vi "FPGA-Main.vi"() -> ()   [LabVIEW 2019]
uses:
  <vilib>/rvi/Emulation/niFpgaGetClockAttributes.vi
  <vilib>/rvi/Emulation/niFpgaSctlEmulationGetInTimedLoop.vi
  <vilib>/rvi/Emulation/niFpgaEmulationReportErrorSimple.vi
  <vilib>/rvi/eio/common/nirviEmuTemplateMethod_errors.vi
  <vilib>/rvi/Emulation/niFpgaEmulationIsFPGAContextNoSignature.vi
  <vilib>/rvi/errors/niFpgaSetErrorForExecOnDevCompSimple.vi
  <vilib>/rvi/eio/common/nirviEmuReportErrorAndStop.vi
  <vilib>/rvi/DataTransferAndStorage/Container/Common/niFpgaContainerGetUniqueNameForEmu.vi
  <vilib>/rvi/FIFO/Fifo_Resource/nirvififoEmulationSetSize.vi
  <vilib>/rvi/FIFO/Fifo_Resource/nirviFifoEmulationQueueMgr.vi
  <instcachedir>/0/nirviFifoEmulationQueueMgr_E5CAEC123FF24DC58D834DCA3CDAA9B5.lvgen/nirviFifoEmulationQueueMgr_E5CAEC123FF24DC58D834DCA3CDAA9B5_006.vi
  <vilib>/rvi/FIFO/Fifo_Resource/nirvififoEmulationDetermineInputValidOut.vi
  <vilib>/rvi/FIFO/Fifo_Resource/nirvififoEmulationCreateLock.vi
  <vilib>/rvi/Emulation/niFpgaProcessEmulError.vi
  <vilib>/rvi/FIFO/Fifo_Resource/nirvififoEmulationObtainLock.vi
  <vilib>/rvi/FIFO/Fifo_Resource/nirvififoEmulationReleaseLock.vi
  <vilib>/rvi/occurrence/nirviWaitOnOccurrenceBase.vi
  <vilib>/rvi/errors/nirviReportUnexpectedCaseInternalError.vi
  <vilib>/rvi/errors/nirviReportUnexpectedCaseInternalError (U32).vi
  <vilib>/rvi/Emulation/niFpgaCriticalErrorInLSC.vi
  <vilib>/Utility/error.llb/Clear Errors.vi
  <vilib>/rvi/interface/RandomDataEmulation/niFpgaRandomDataHandleErrors.vi
  <vilib>/rvi/interface/RandomDataEmulation/nirviRandomDataMultiElementFPGAFIFO.vi
  <instcachedir>/0/nirviRandomDataMultiElementFPGAFIFO_1ED88BA00AC641F388A9B1FAA20E354D.lvgen/nirviRandomDataMultiElementFPGAFIFO_1ED88BA00AC641F388A9B1FAA20E354D_004.vi
  <vilib>/eio/EIONode/EIONode.xnode
  <vilib>/rvi/DataTransferAndStorage/Container/XNode/niFpgaContainer.xnode
  <vilib>/rvi/FIFO/Fifo_Resource/nirvififoEmulationWrite.vi
  <vilib>/rvi/FIFO/Fifo_Resource/nirvififoEmulationRead.vi
  <vilib>/rvi/interface/RandomDataEmulation/nirviRandomDataFpgaReadWriteTemplate.vi
  <vilib>/rvi/Analysis/measure/butterworth/XNode/niFpgaButterworthFilter.xnode
  <vilib>/rvi/interface/RandomDataEmulation/nirviRandomDataFpgaMultiElementTemplate.vi
panel:
  out "超时？ 2":bool
  out "超时？":bool
  in  "Count(uSec)":u32=10 caption="计数器(uSec)"
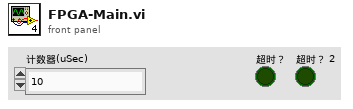
[diagram p1: front panel]
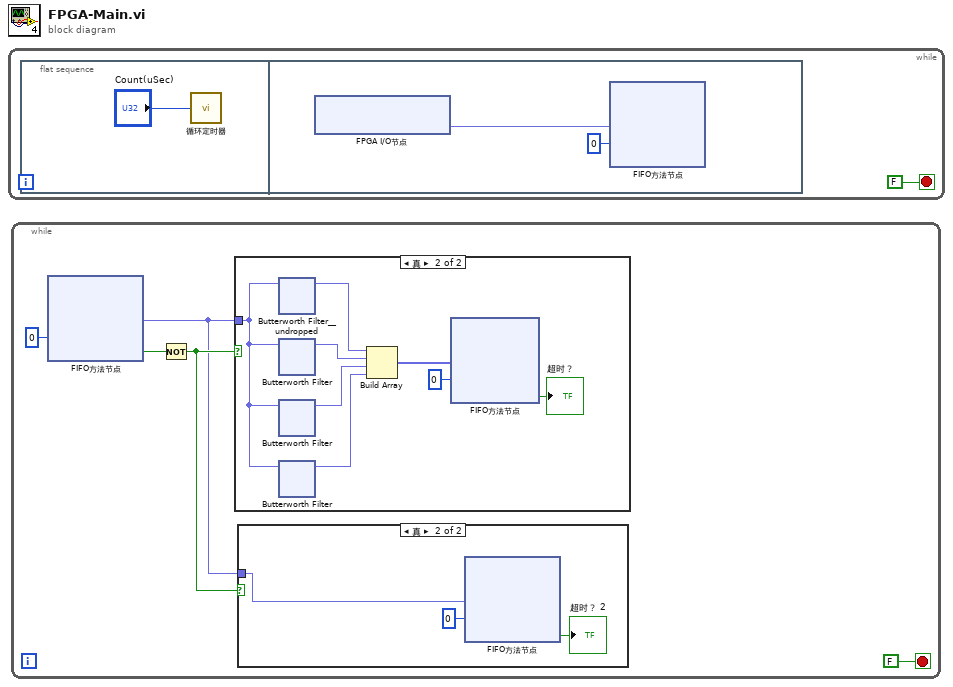
[diagram p0: block diagram]
diagram:
  n1 = while {
    stop <- FALSE stop-if-true
    n2 = flat-sequence {
      frame #0 {
        n3 = call "循环定时器"("Count(uSec)"="Count(uSec)") -> ()  [unwired: 1 out]
      }
      frame #1 {
        n4 = xnode "FPGA I/O节点"() -> ("ConnectorB/AI0"=w4:fxp<+/-,24,5>)  [unwired: 1 in, 1 out]
        n5 = xnode ("FIFO方法节点")("元素"=w4, "超时"=0) -> ()  [unwired: 1 in, 2 out]
      }
    }
  }
  n6 = while {
    stop <- FALSE stop-if-true
    n7 = xnode ("FIFO方法节点")("超时"=0) -> ("元素"=w6:fxp<+/-,24,5>, "超时？"=w9:bool)  [unwired: 1 in, 1 out]
    n8 = Not(x=w9) -> (.not. x?=w7:bool)
    n9 = case shown="真" w7 {
      tunnel: w6 -> [_ w20]
      frame False {
      }
      frame True {
        n10 = xnode "Butterworth Filter__undropped"("输入数据"=w20) -> ("输出数据"=w19:fxp<+/-,24,5>)  [unwired: 2 in]
        n11 = xnode "Butterworth Filter"("输入数据"=w20) -> ("输出数据"=w18:fxp<+/-,24,5>)  [unwired: 2 in]
        n12 = xnode "Butterworth Filter"("输入数据"=w20) -> ("输出数据"=w17:fxp<+/-,24,5>)  [unwired: 2 in]
        n13 = xnode "Butterworth Filter"("输入数据"=w20) -> ("输出数据"=w16:fxp<+/-,24,5>)  [unwired: 2 in]
        n14 = Build Array(w19, w18, w17, w16) -> (w15:fxp<+/-,24,5>[])
        n15 = xnode ("FIFO方法节点")("元素"=w15, "超时"=0) -> ("超时？"=→"超时？":bool)  [unwired: 1 in, 1 out]
      }
    }
    n16 = case shown="真" w7 {
      tunnel: w6 -> [_ w12]
      frame False {
      }
      frame True {
        n17 = xnode ("FIFO方法节点")("元素"=w12, "超时"=0) -> ("超时？"=→"超时？ 2":bool)  [unwired: 1 in, 1 out]
      }
    }
  }
